vi "Monitor MC data.vi"(7 "IP/condition":T1(ring), 8 "error in (no error)":errorcluster, 9 "Lower limits [um]":dbl, 10 "Upper limits [um]":dbl, 11 "MC data IN":dbl[](array[numeric])) -> (0 "error out":errorcluster, 1 "RESTART MC":bool, 2 "Reset Transition Status":T1(ring), 3 "Status":T2(ring))   [LabVIEW 2020]
uses:
  Typedefs/fgv_actions.ctl
  Global Variables/General Globals.vi
panel:
  out "User reset":bool
  out "ms":u32
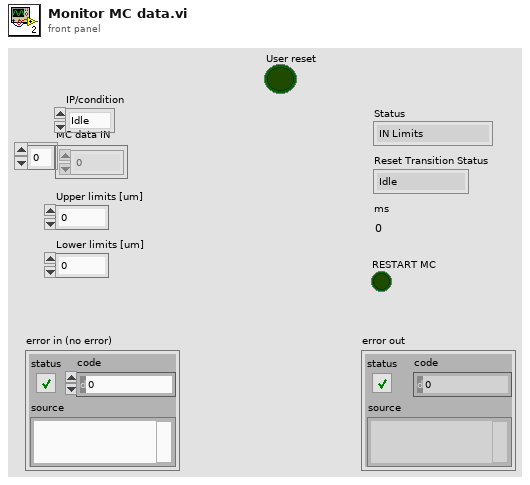
[diagram p1: front panel]
types:
  T1 = enum16{"Idle", "Stop MC Tracking", "Wait process", "Monitor error", "Restart MC Tracking"}
  T2 = enum16{"IN Limits", "X/Y Exceeded", "Z Exceeded", "X/Y & Z Exceeded"}
  T3 = typedef "fgv_actions.ctl" = enum16{"Get", "Set"}
  T4 = enum16{"Idle", "Stop Tracking", "Start Tracking"}
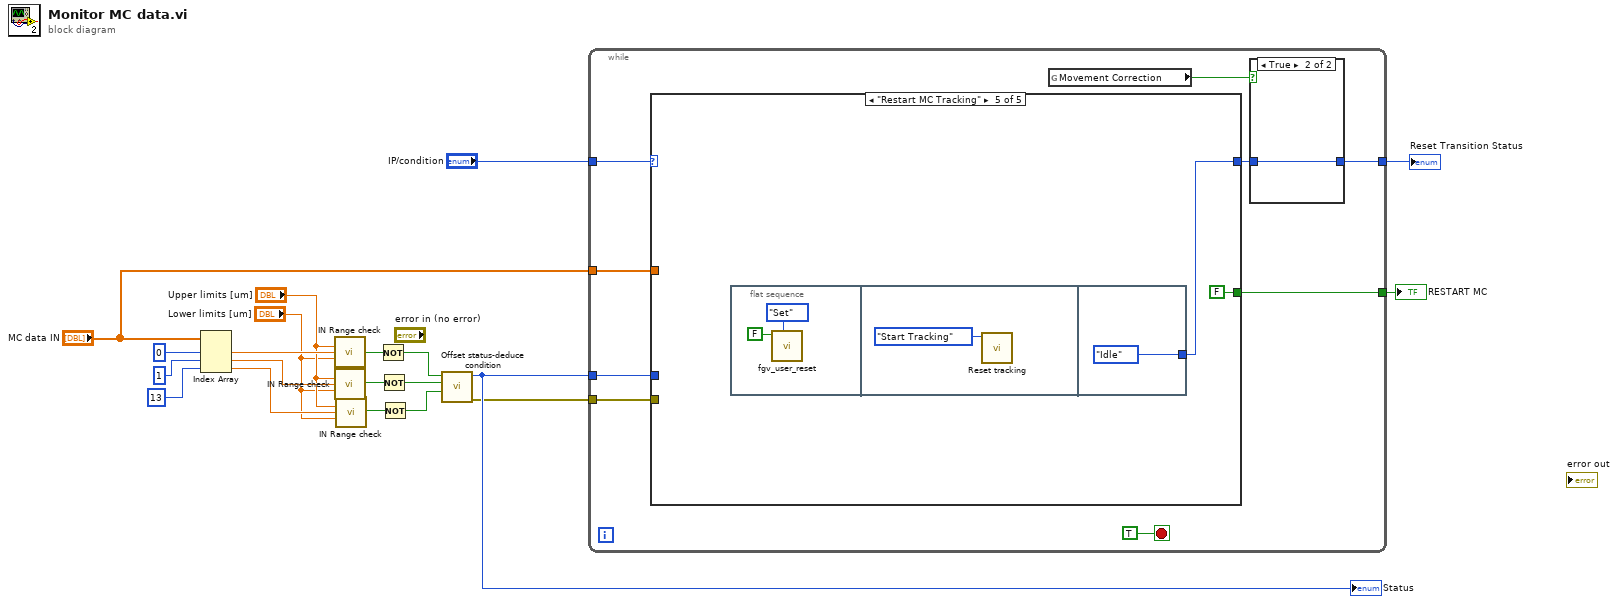
[diagram p0: block diagram]
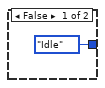
[diagram p2: hidden frame]
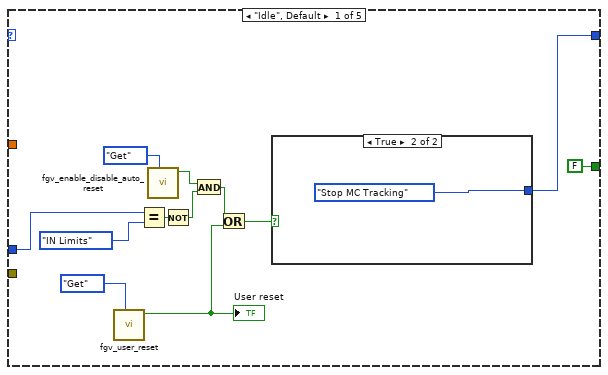
[diagram p3: hidden frame]
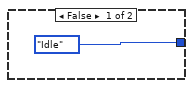
[diagram p4: hidden frame]
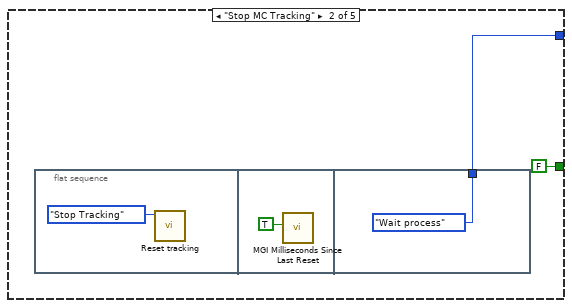
[diagram p5: hidden frame]
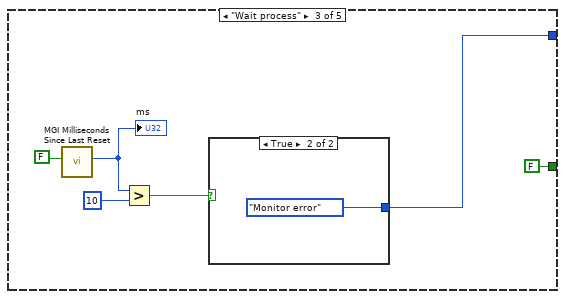
[diagram p6: hidden frame]
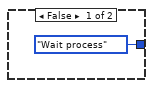
[diagram p7: hidden frame]
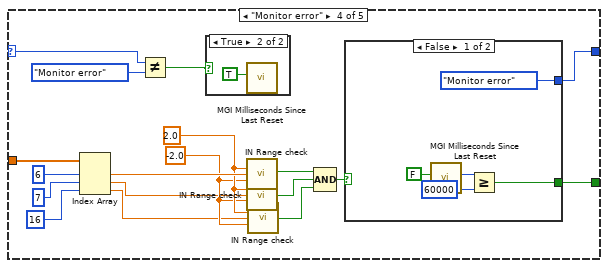
[diagram p8: hidden frame]
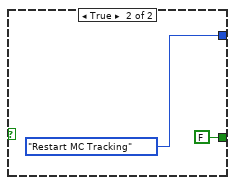
[diagram p10: hidden frame]
diagram:
  n1 = Index Array(array="MC data IN", index #1=0 ("index"), index #2=1 ("index"), index #3=13 ("index")) -> (element #1=w17:dbl, element #2=w16:dbl, element #3=w15:dbl)
  n2 = call "IN Range check.vi"("UL"="Upper limits [um]", "Data Point"=w17, "LL"="Lower limits [um]") -> ("In range ?"=w8:bool)  [unwired: 12 in]
  n3 = call "IN Range check.vi"("UL"="Upper limits [um]", "Data Point"=w16, "LL"="Lower limits [um]") -> ("In range ?"=w5:bool)  [unwired: 12 in]
  n4 = call "IN Range check.vi"("UL"="Upper limits [um]", "Data Point"=w15, "LL"="Lower limits [um]") -> ("In range ?"=w4:bool)  [unwired: 12 in]
  n5 = Not(x=w8) -> (.not. x?=w7:bool)
  n6 = Not(x=w5) -> (.not. x?=w6:bool)
  n7 = Not(x=w4) -> (.not. x?=w3:bool)
  n8 = call "Offset status-deduce condition.vi"("Z_offset"=w3, "Y_offset"=w6, "X_offset"=w7) -> ("error out"=w10:errorcluster, "Status"=w12:T2)  [unwired: 7 in]
  "Status" <- w12
  n9 = while {
    tunnel: w12 -> [w29]
    tunnel: w10 -> [w26]
    tunnel: "MC data IN" -> [w25]
    tunnel: [w21] -> w1
    tunnel: "IP/condition" -> [w27]
    tunnel: [w23] -> w2
    stop <- TRUE stop-if-true
    n10 = case shown="\"Restart MC Tracking\"" w27 {
      selector: w27 -> [_ _ _ w62 _]
      tunnel: w29 -> [w43 _ _ _ _]
      tunnel: [w41 w46 w56 w63 w86] -> w22
      tunnel: w26 -> [_ _ _ _ _]
      tunnel: w25 -> [_ _ _ w73 _]
      tunnel: [FALSE FALSE FALSE w59 FALSE] -> w21
      frame "Idle", Default {
        n11 = call "fgv_user_reset.vi"("FGV Actions"=fgv_actions."Get") -> ("User reset"=w37:bool)  [unwired: 9 in, 1 out]
        "User reset" <- w37
        n12 = Equal?(x=w43, y=T2."IN Limits") -> (x = y?=w38:bool)
        n13 = call "fgv_enable_disable_auto_reset.vi"("FGV Actions"=fgv_actions."Get") -> ("Auto reset"=w34:bool)  [unwired: 9 in, 1 out]
        n14 = Not(x=w38) -> (.not. x?=w33:bool)
        n15 = And(x=w34, y=w33) -> (x .and. y?=w32:bool)
        n16 = Or(x=w32, y=w37) -> (x .or. y?=w36:bool)
        n17 = case shown="True" w36 {
          tunnel: [T1."Idle" ("Enum") T1."Stop MC Tracking" ("Enum")] -> w41
          frame False {
          }
          frame True {
          }
        }
      }
      frame "Stop MC Tracking" {
        n18 = flat-sequence {
          tunnel: [T1."Wait process" ("Enum")] -> w46
          frame #0 {
            n19 = call "Reset tracking.vi"("Stop Tracking"=T4."Stop Tracking") -> ()  [unwired: 11 in]
          }
          frame #1 {
            n20 = call <userlib>:"MGI Milliseconds Since Last Reset.vi"("Reset (F)"=TRUE) -> ()  [unwired: 5 in, 2 out]
          }
          frame #2 {
          }
        }
      }
      frame "Wait process" {
        n21 = call <userlib>:"MGI Milliseconds Since Last Reset.vi"("Reset (F)"=FALSE) -> ("ms"=w54:u32)  [unwired: 5 in, 1 out]
        "ms" <- w54
        n22 = Greater?(x=w54, y=u32 10) -> (0:w52:bool)
        n23 = case shown="True" w52 {
          tunnel: [T1."Wait process" ("Enum") T1."Monitor error" ("Enum")] -> w56
          frame False {
          }
          frame True {
          }
        }
      }
      frame "Monitor error" {
        w70 = -2.0 ("LL")
        w71 = 2.0 ("UL")
        n24 = Index Array(array=w73, index #1=6 ("index"), index #2=7 ("index"), index #3=16 ("index")) -> (element #1=w72:dbl, element #2=w69:dbl, element #3=w68:dbl)
        n25 = Not Equal?(x=w62, y=T1."Monitor error") -> (x != y?=w60:bool)
        n26 = case shown="True" w60 {
          frame False {
          }
          frame True {
            n27 = call <userlib>:"MGI Milliseconds Since Last Reset.vi"("Reset (F)"=TRUE) -> ()  [unwired: 5 in, 2 out]
          }
        }
        n28 = call "IN Range check.vi"("UL"=w71, "Data Point"=w72, "LL"=w70) -> ("In range ?"=w67:bool)  [unwired: 12 in]
        n29 = call "IN Range check.vi"("UL"=w71, "Data Point"=w69, "LL"=w70) -> ("In range ?"=w66:bool)  [unwired: 12 in]
        n30 = call "IN Range check.vi"("UL"=w71, "Data Point"=w68, "LL"=w70) -> ("In range ?"=w65:bool)  [unwired: 12 in]
        n31 = Compound Arithmetic op=AND(w67, w66, w65) -> (w64:bool)
        n32 = case shown="False" w64 {
          tunnel: [T1."Monitor error" ("Enum") T1."Restart MC Tracking" ("Enum")] -> w63
          tunnel: [w78 FALSE] -> w59
          frame False {
            n33 = call <userlib>:"MGI Milliseconds Since Last Reset.vi"("Reset (F)"=FALSE) -> ("ms"=w80:u32)  [unwired: 5 in, 1 out]
            n34 = Greater Or Equal?(x=w80, y=u32 60000) -> (x >= y?=w78:bool)
          }
          frame True {
          }
        }
      }
      frame "Restart MC Tracking" {
        n35 = flat-sequence {
          tunnel: [T1."Idle" ("Enum")] -> w86
          frame #0 {
            n36 = call "fgv_user_reset.vi"("FGV Actions"=fgv_actions."Set", "User reset"=FALSE) -> ()  [unwired: 8 in, 2 out]
          }
          frame #1 {
            n37 = call "Reset tracking.vi"("Stop Tracking"=T4."Start Tracking") -> ()  [unwired: 11 in]
          }
          frame #2 {
          }
        }
      }
    }
    n38 = global read "General Globals.vi" "Movement Correction"() -> (w24:bool)
    n39 = case shown="True" w24 {
      tunnel: [T1."Idle" ("Enum") w31] -> w23
      tunnel: w22 -> [_ w31]
      frame False {
      }
      frame True {
      }
    }
  }
  "Reset Transition Status" <- w2
  "RESTART MC" <- w1
